vi "Write dc.vi"(8 "error in (no error)":errorcluster, 10 "dc":dbl, 11 "Change DC in":refnum<class "Change DC MSG.lvclass">) -> (0 "error out":errorcluster, 3 "Change DC out":refnum<class "Change DC MSG.lvclass">)   [LabVIEW 2014, in "eCRDS Library.lvlib" / "Change DC MSG.lvclass"]
uses:
  Change DC MSG.lvclass
  Change DC MSG.lvclass/Change DC MSG.ctl
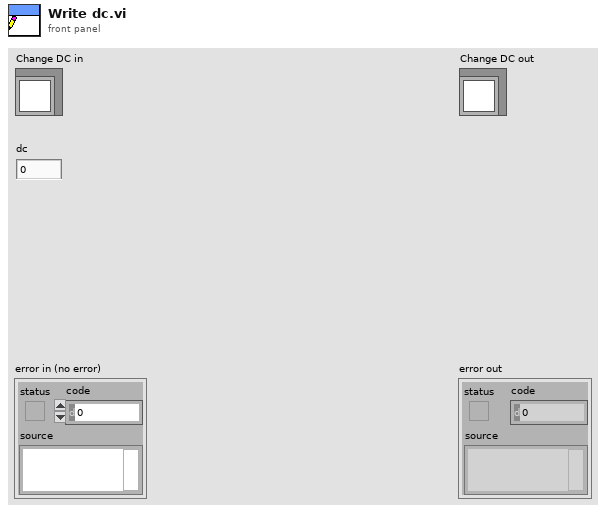
[diagram p1: front panel]
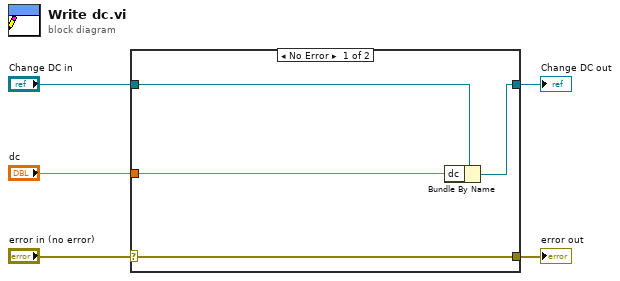
[diagram p0: block diagram]
diagram:
  n1 = case shown="No Error" "error in (no error)" {
    selector: "error in (no error)" -> [w9 w10]
    tunnel: [w9 w10] -> w4
    tunnel: [w7 w11] -> w2
    tunnel: "Change DC in" -> [w8 w11]
    tunnel: "dc" -> [w6 _]
    frame No Error {
      n2 = Bundle By Name(cluster=w8, "dc"=w6) -> (w7:refnum<class "Change DC MSG.lvclass">)
    }
    frame Error {
    }
  }
  "error out" <- w4
  "Change DC out" <- w2
